vi "draw_block.vi"(9 "input plate":picture, 10 "position":cluster{"x":u16, "y":u16}, 11 "block_type":enum16{"line", "block", "T", "L", "rev_L"}(ring)) -> (3 "output":picture)   [LabVIEW 2024]
panel:
  in  "block_dire":dbl
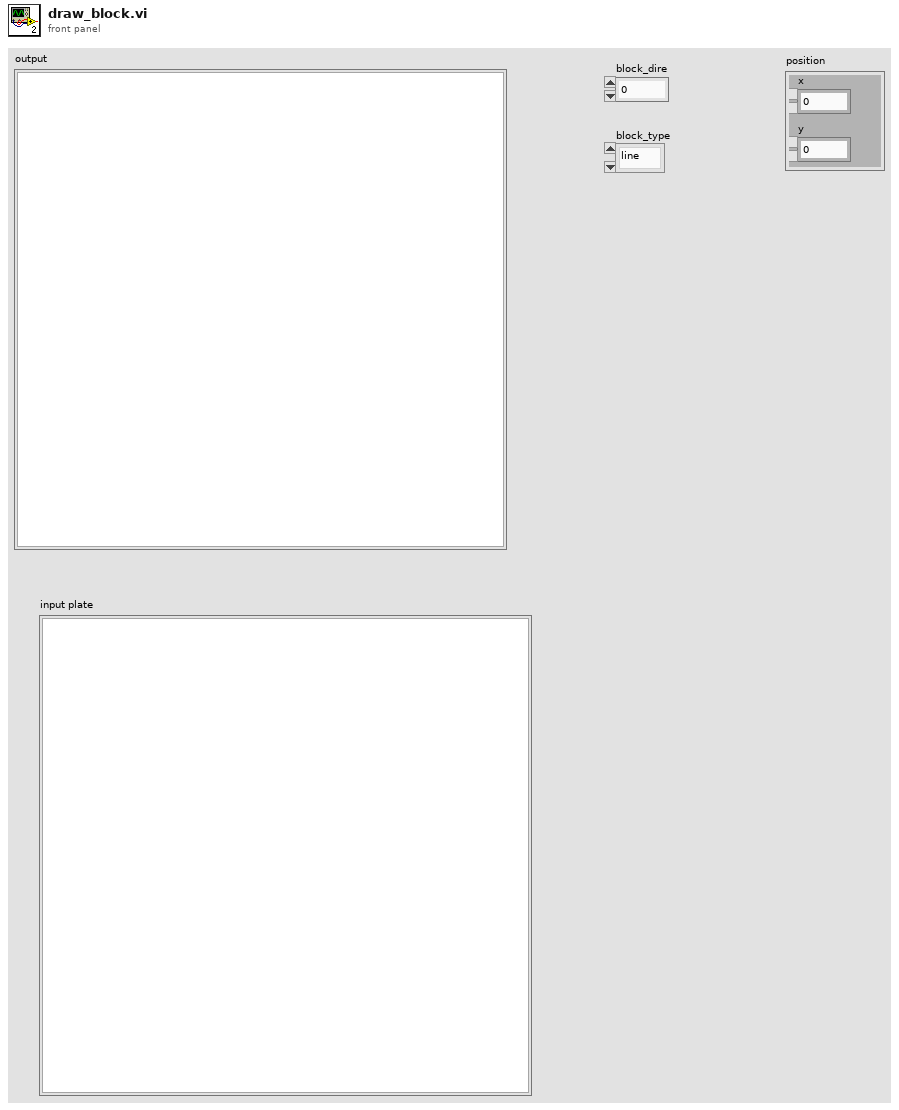
[diagram p1: front panel]
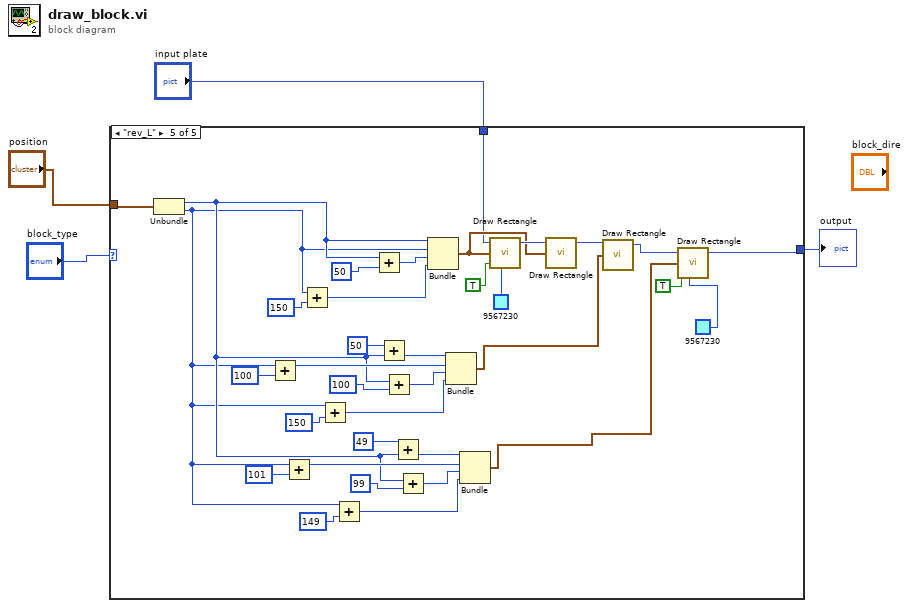
[diagram p0: block diagram]
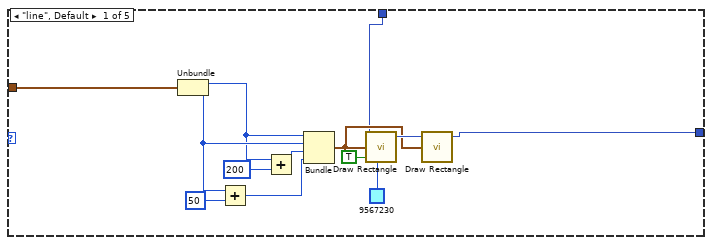
[diagram p2: hidden frame]
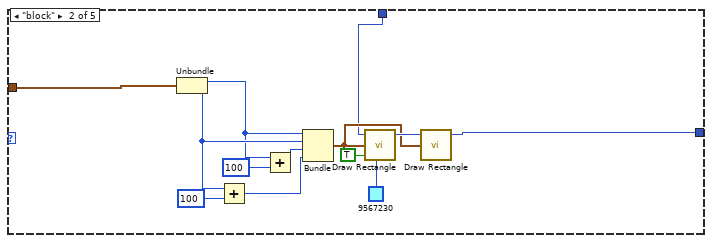
[diagram p3: hidden frame]
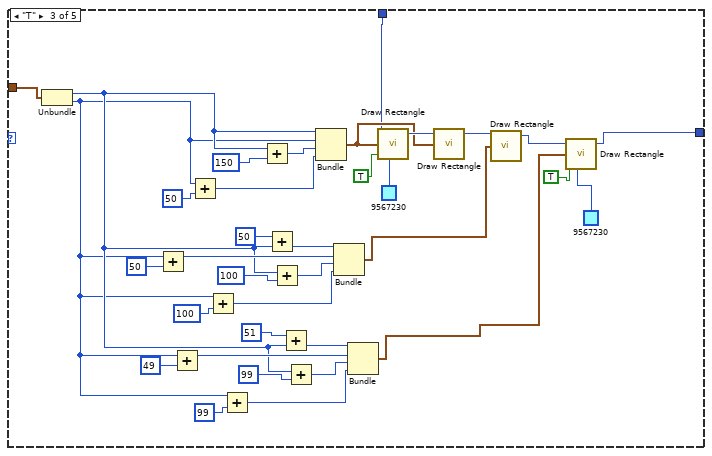
[diagram p4: hidden frame]
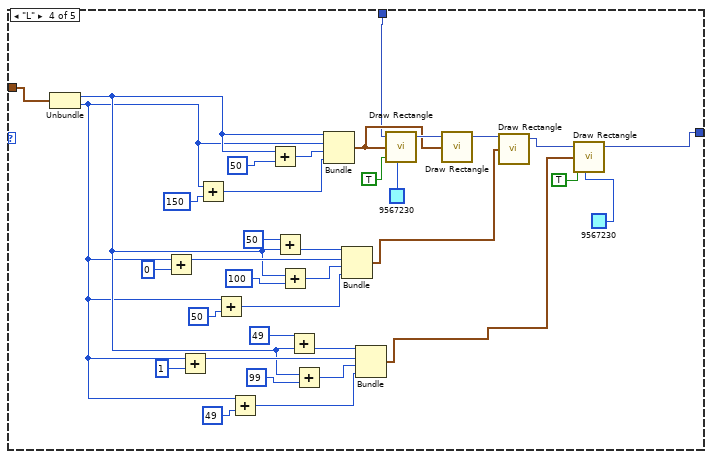
[diagram p5: hidden frame]
diagram:
  n1 = case shown="\"rev_L\"" "block_type" {
    tunnel: [w8 w19 w32 w67 w102] -> w3
    tunnel: "position" -> [w6 w20 w57 w68 w103]
    tunnel: "input plate" -> [w5 w18 w31 w66 w101]
    frame "line", Default {
      n2 = Unbundle(w6) -> ("x"=w14:u16, "y"=w17:u16)
      n3 = Add(x=w17, y=u16 50) -> (x+y=w15:u16)
      n4 = Add(x=w14, y=u16 200) -> (x+y=w12:u16)
      n5 = Bundle("x"=w14, "y"=w17, w12, w15) -> (w7:cluster{"x":u16, "y":u16, u16, u16})  [unwired: 1 in]
      n6 = call <vilib>:"Draw Rectangle.vi"("picture"=w5, "rect"=w7, "fill?(F)"=TRUE, "color(black)"=u32 9567230) -> ("new picture"=w9:picture)  [unwired: 5 in]
      n7 = call <vilib>:"Draw Rectangle.vi"("picture"=w9, "rect"=w7) -> ("new picture"=w8:picture)  [unwired: 7 in]
    }
    frame "block" {
      n8 = Unbundle(w20) -> ("x"=w28:u16, "y"=w30:u16)
      n9 = Add(x=w30, y=u16 100) -> (x+y=w29:u16)
      n10 = Add(x=w28, y=u16 100) -> (x+y=w27:u16)
      n11 = Bundle("x"=w28, "y"=w30, w27, w29) -> (w25:cluster{"x":u16, "y":u16, u16, u16})  [unwired: 1 in]
      n12 = call <vilib>:"Draw Rectangle.vi"("picture"=w18, "rect"=w25, "fill?(F)"=TRUE, "color(black)"=u32 9567230) -> ("new picture"=w26:picture)  [unwired: 5 in]
      n13 = call <vilib>:"Draw Rectangle.vi"("picture"=w26, "rect"=w25) -> ("new picture"=w19:picture)  [unwired: 7 in]
    }
    frame "T" {
      n14 = Unbundle(w57) -> ("x"=w38:u16, "y"=w37:u16)
      n15 = Add(x=w37, y=u16 50) -> (x+y=w50:u16)
      n16 = Add(x=w37, y=u16 49) -> (x+y=w45:u16)
      n17 = Add(x=w37, y=u16 50) -> (x+y=w65:u16)
      n18 = Add(x=w37, y=u16 100) -> (x+y=w53:u16)
      n19 = Add(x=w37, y=u16 99) -> (x+y=w42:u16)
      n20 = Add(x=w38, y=u16 150) -> (x+y=w64:u16)
      n21 = Add(x=u16 50, y=w38) -> (x+y=w52:u16)
      n22 = Add(x=w38, y=u16 100) -> (x+y=w54:u16)
      n23 = Add(x=u16 51, y=w38) -> (x+y=w43:u16)
      n24 = Add(x=w38, y=u16 99) -> (x+y=w41:u16)
      n25 = Bundle("x"=w38, "y"=w37, w64, w65) -> (w62:cluster{"x":u16, "y":u16, u16, u16})  [unwired: 1 in]
      n26 = Bundle(w52, w50, w54, w53) -> (w36:cluster{u16, u16, u16, u16})  [unwired: 1 in]
      n27 = Bundle(w43, w45, w41, w42) -> (w35:cluster{u16, u16, u16, u16})  [unwired: 1 in]
      n28 = call <vilib>:"Draw Rectangle.vi"("picture"=w31, "rect"=w62, "fill?(F)"=TRUE, "color(black)"=u32 9567230) -> ("new picture"=w63:picture)  [unwired: 5 in]
      n29 = call <vilib>:"Draw Rectangle.vi"("picture"=w63, "rect"=w62) -> ("new picture"=w34:picture)  [unwired: 7 in]
      n30 = call <vilib>:"Draw Rectangle.vi"("picture"=w34, "rect"=w36) -> ("new picture"=w33:picture)  [unwired: 7 in]
      n31 = call <vilib>:"Draw Rectangle.vi"("picture"=w33, "rect"=w35, "fill?(F)"=TRUE, "color(black)"=u32 9567230) -> ("new picture"=w32:picture)  [unwired: 5 in]
    }
    frame "L" {
      n32 = Unbundle(w68) -> ("x"=w88:u16, "y"=w87:u16)
      n33 = Add(x=w87, y=u16 0) -> (x+y=w93:u16)
      n34 = Add(x=w87, y=u16 1) -> (x+y=w92:u16)
      n35 = Add(x=w87, y=u16 150) -> (x+y=w100:u16)
      n36 = Add(x=w87, y=u16 50) -> (x+y=w95:u16)
      n37 = Add(x=w87, y=u16 49) -> (x+y=w90:u16)
      n38 = Add(x=w88, y=u16 50) -> (x+y=w99:u16)
      n39 = Add(x=u16 50, y=w88) -> (x+y=w94:u16)
      n40 = Add(x=w88, y=u16 100) -> (x+y=w96:u16)
      n41 = Add(x=u16 49, y=w88) -> (x+y=w91:u16)
      n42 = Add(x=w88, y=u16 99) -> (x+y=w89:u16)
      n43 = Bundle("x"=w88, "y"=w87, w99, w100) -> (w97:cluster{"x":u16, "y":u16, u16, u16})  [unwired: 1 in]
      n44 = Bundle(w94, w93, w96, w95) -> (w86:cluster{u16, u16, u16, u16})  [unwired: 1 in]
      n45 = Bundle(w91, w92, w89, w90) -> (w85:cluster{u16, u16, u16, u16})  [unwired: 1 in]
      n46 = call <vilib>:"Draw Rectangle.vi"("picture"=w66, "rect"=w97, "fill?(F)"=TRUE, "color(black)"=u32 9567230) -> ("new picture"=w98:picture)  [unwired: 5 in]
      n47 = call <vilib>:"Draw Rectangle.vi"("picture"=w98, "rect"=w97) -> ("new picture"=w84:picture)  [unwired: 7 in]
      n48 = call <vilib>:"Draw Rectangle.vi"("picture"=w84, "rect"=w86) -> ("new picture"=w83:picture)  [unwired: 7 in]
      n49 = call <vilib>:"Draw Rectangle.vi"("picture"=w83, "rect"=w85, "fill?(F)"=TRUE, "color(black)"=u32 9567230) -> ("new picture"=w67:picture)  [unwired: 5 in]
    }
    frame "rev_L" {
      n50 = Unbundle(w103) -> ("x"=w123:u16, "y"=w122:u16)
      n51 = Add(x=w122, y=u16 100) -> (x+y=w128:u16)
      n52 = Add(x=w122, y=u16 101) -> (x+y=w127:u16)
      n53 = Add(x=w122, y=u16 150) -> (x+y=w135:u16)
      n54 = Add(x=w122, y=u16 150) -> (x+y=w130:u16)
      n55 = Add(x=w122, y=u16 149) -> (x+y=w125:u16)
      n56 = Add(x=w123, y=u16 50) -> (x+y=w134:u16)
      n57 = Add(x=u16 50, y=w123) -> (x+y=w129:u16)
      n58 = Add(x=w123, y=u16 100) -> (x+y=w131:u16)
      n59 = Add(x=u16 49, y=w123) -> (x+y=w126:u16)
      n60 = Add(x=w123, y=u16 99) -> (x+y=w124:u16)
      n61 = Bundle("x"=w123, "y"=w122, w134, w135) -> (w132:cluster{"x":u16, "y":u16, u16, u16})  [unwired: 1 in]
      n62 = Bundle(w129, w128, w131, w130) -> (w121:cluster{u16, u16, u16, u16})  [unwired: 1 in]
      n63 = Bundle(w126, w127, w124, w125) -> (w120:cluster{u16, u16, u16, u16})  [unwired: 1 in]
      n64 = call <vilib>:"Draw Rectangle.vi"("picture"=w101, "rect"=w132, "fill?(F)"=TRUE, "color(black)"=u32 9567230) -> ("new picture"=w133:picture)  [unwired: 5 in]
      n65 = call <vilib>:"Draw Rectangle.vi"("picture"=w133, "rect"=w132) -> ("new picture"=w119:picture)  [unwired: 7 in]
      n66 = call <vilib>:"Draw Rectangle.vi"("picture"=w119, "rect"=w121) -> ("new picture"=w118:picture)  [unwired: 7 in]
      n67 = call <vilib>:"Draw Rectangle.vi"("picture"=w118, "rect"=w120, "fill?(F)"=TRUE, "color(black)"=u32 9567230) -> ("new picture"=w102:picture)  [unwired: 5 in]
    }
  }
  "output" <- w3
